vi "module-07-exercise-7-2-ENUM-template.vi"() -> ()   [LabVIEW 2019]
uses:
  DiscShooterState_ENUM.ctl
  <vilib>/Rock Robotics/WPI/ThirdParty/JAS_Junk/TrajLib/Trajectory_Library.lvlib
panel:
  out "DiscShootState":T1
  in  "Have Disc \nLimit Switch Sensor":bool
  in  "Battery Voltage":dbl=11.0 min=0.0 max=14.0 step=0.1
  in  "Driver Shoot Button":bool
  in  "Driver Cancel Button":bool
  out "Shoot Request":bool
  out "Digital State Chart":cluster{dbl, dbl, dbl, dbl, dbl, dbl}(graph)
  out "Ready to Shoot":bool
  out "Engage Solenoid":bool
  out "Shooting Motor":bool
  out "State":i32
  out "Current Timer Value":dbl format="%20.3f"
  out "Cur Time":dbl format="%20.3f"
  # "Training Exercise 7-2 Template\nDisc Shooter"
  # "F1"
  # "F2"
  # "F3"
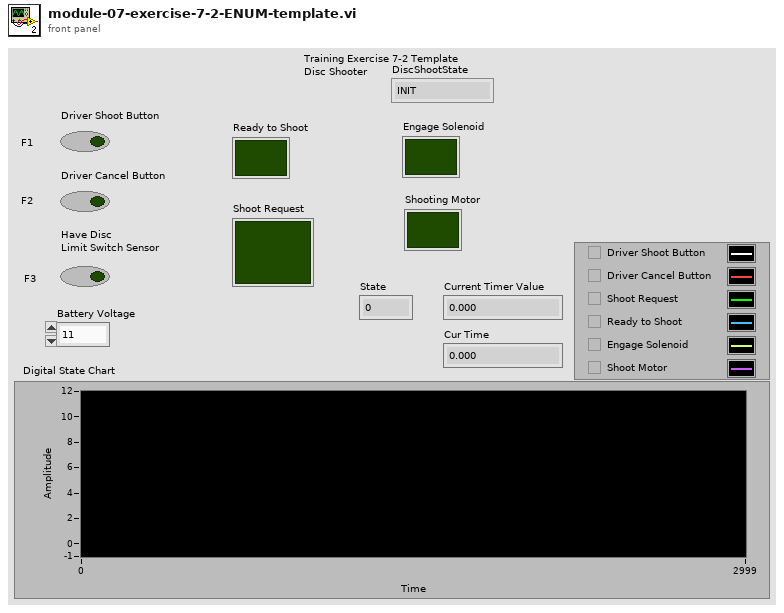
[diagram p1: front panel]
types:
  T1 = typedef "DiscShooterState_ENUM.ctl" = enum16{"INIT"}
  T2 = typedef "Trajectory_Library.lvlib/TIMER.ctl" = cluster{"StartTime":dbl, "Accumulated TIme":dbl, "Running":bool, "semaphore":T3}
  T3 = typedef "Semaphore RefNum" = refnum<k1>
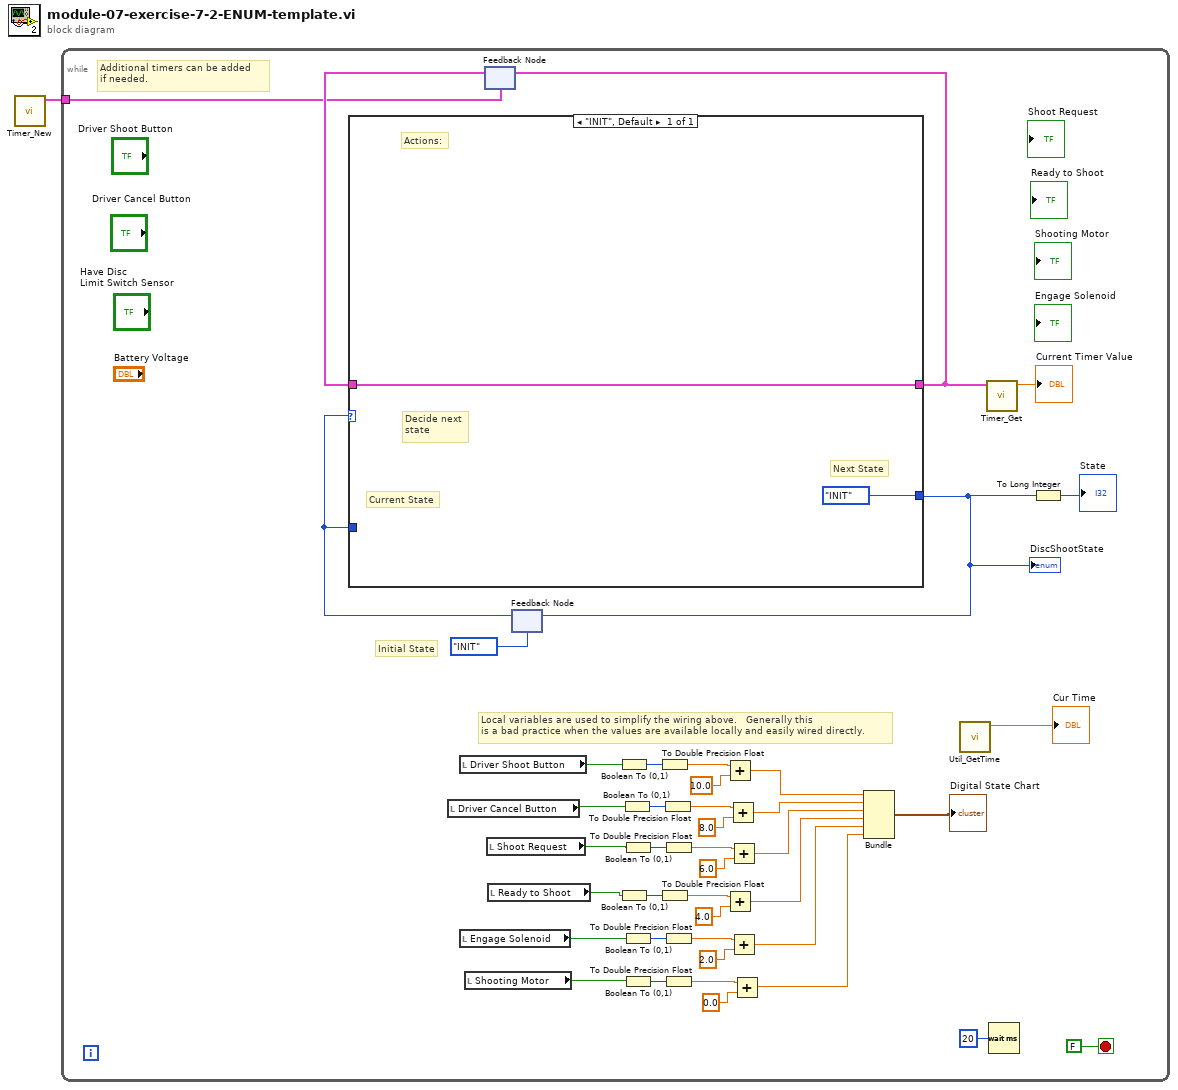
[diagram p0: block diagram]
diagram:
  n1 = call <vilib>:"Timer_New.vi"() -> ("TIMER"=w1:T2)  [unwired: 11 in]
  n2 = while {
    tunnel: w1 -> [w10]
    stop <- FALSE stop-if-true
    # "Additional timers can be added \nif needed."
    # "Initial State"
    # "Local variables are used to simplify the wiring above.   Generally this\nis a bad practice when the values are available locally and easily wired directly."
    n3 = local read "Driver Cancel Button"() -> (w6:bool)
    n4 = local read "Driver Shoot Button"() -> (w5:bool)
    n5 = local read "Engage Solenoid"() -> (w15:bool)
    n6 = local read "Shooting Motor"() -> (w16:bool)
    n7 = feedback #1(w10) -> (w12:T2)
    n8 = local read "Shoot Request"() -> (w14:bool)
    n9 = local read "Ready to Shoot"() -> (w13:bool)
    n10 = feedback #2(DiscShooterState_ENUM."INIT" ("DiscShootState")) -> (w11:T1)
    n11 = case shown="\"INIT\", Default" w11 {
      tunnel: [DiscShooterState_ENUM."INIT" ("DiscShootState")] -> w2
      tunnel: [w45] -> w8
      tunnel: w12 -> [w45]
      tunnel: w11 -> [_]
      frame "INIT", Default {
        # "Decide next\nstate"
        # "Current State"
        # "Next State"
        # "Actions:"
      }
    }
    "DiscShootState" <- w2
    n12 = feedback-in #1(w8) -> ()
    n13 = feedback-in #2(w2) -> ()
    n14 = Boolean To (0,1)(Boolean=w5) -> (0, 1=w41:i16)
    n15 = Boolean To (0,1)(Boolean=w13) -> (0, 1=w39:i16)
    n16 = Boolean To (0,1)(Boolean=w6) -> (0, 1=w36:i16)
    n17 = Boolean To (0,1)(Boolean=w14) -> (0, 1=w33:i16)
    n18 = Boolean To (0,1)(Boolean=w15) -> (0, 1=w30:i16)
    n19 = Boolean To (0,1)(Boolean=w16) -> (0, 1=w27:i16)
    n20 = To Double Precision Float(number=w41) -> (double precision float=w18:dbl)
    n21 = To Double Precision Float(number=w39) -> (double precision float=w38:dbl)
    n22 = To Double Precision Float(number=w36) -> (double precision float=w35:dbl)
    n23 = To Double Precision Float(number=w33) -> (double precision float=w32:dbl)
    n24 = To Double Precision Float(number=w30) -> (double precision float=w29:dbl)
    n25 = To Double Precision Float(number=w27) -> (double precision float=w26:dbl)
    n26 = Add(x=w18, y=10.0) -> (x+y=w17:dbl)
    n27 = Add(x=w38, y=4.0) -> (x+y=w21:dbl)
    n28 = Add(x=w35, y=8.0) -> (x+y=w23:dbl)
    n29 = Add(x=w32, y=6.0) -> (x+y=w22:dbl)
    n30 = Add(x=w29, y=2.0) -> (x+y=w25:dbl)
    n31 = Add(x=w26, y=0.0) -> (x+y=w24:dbl)
    n32 = Bundle(w17, w23, w22, w21, w25, w24) -> (→"Digital State Chart":cluster{dbl, dbl, dbl, dbl, dbl, dbl})  [unwired: 1 in]
    n33 = call <vilib>:"Util_GetTime.vi"() -> ("FPGA_Time_Seconds"=→"Cur Time":dbl)  [unwired: 10 in, 1 out]
    n34 = call <vilib>:"Timer_Get.vi"("TIMER"=w8) -> ("CurrentTImer"=→"Current Timer Value":dbl)  [unwired: 10 in]
    n35 = Wait (ms)(milliseconds to wait=u32 20) -> ()  [unwired: 1 out]
    n36 = To Long Integer(number=w2) -> (32bit integer=→"State":i32)
  }
